vi "Write File Record.vi"(0 "MB session in":refnum<class "MB_Master.lvclass">, 1 "仪器版本":T1, 5 "File Number":u16, 7 "Record Number":u16, 9 "values":u16[](array[numeric]), 11 "error in (no error)":errorcluster) -> (4 "MB session out":refnum<class "MB_Master.lvclass">, 15 "error out":errorcluster)   [LabVIEW 2016, in "斯坦道总氮.lvlib"]
uses:
  <vilib>/Plasmionique/MB Master/MB_Master/MB_Master.lvclass
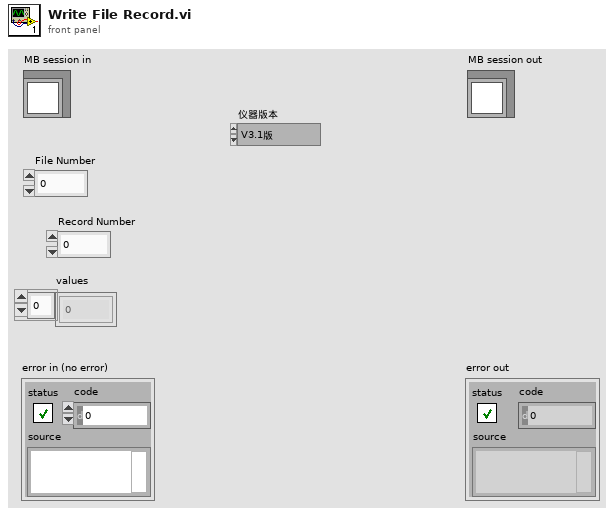
[diagram p1: front panel]
types:
  T1 = typedef "SingleStepTestV3.lvlib/SingleStepTestV3.lvclass/仪器版本.ctl" = enum16{"V3.1版", "V4版", "V3版", "V4.2版"}
  T2 = typedef "MB Master.lvlib/MB_PDU_Cluster.ctl" = cluster{"Function Code":u8, "Data":u8[], "RTU_DataBytes":i32}
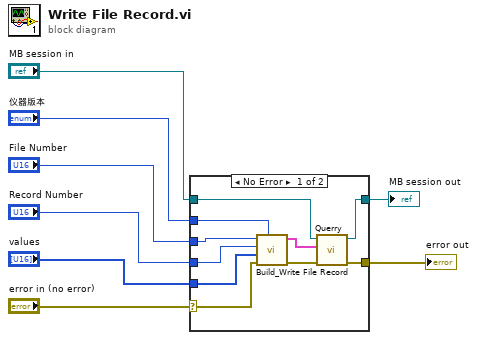
[diagram p0: block diagram]
diagram:
  n1 = case shown="No Error" "error in (no error)" {
    selector: "error in (no error)" -> [w13 w20]
    tunnel: [w17 w20] -> w7
    tunnel: [w18 w19] -> w5
    tunnel: "MB session in" -> [w16 w19]
    tunnel: "File Number" -> [w15 _]
    tunnel: "values" -> [w14 _]
    tunnel: "Record Number" -> [w10 _]
    tunnel: "仪器版本" -> [w9 _]
    frame No Error {
      n2 = call "Build_Write File Record.vi"("File Number"=w15, "Record Number"=w10, "values"=w14, "error in (no error)"=w13, "仪器版本"=w9) -> ("MB_PDU"=w12:T2, "error out"=w11:errorcluster)  [unwired: 4 in]
      n3 = call-dynamic "Querry.vi"("error in (no error)"=w11, "PDU_req"=w12, "MB_Master in"=w16) -> ("error out"=w17:errorcluster, "MB_Master out"=w18:refnum<class "MB_Master.lvclass">)  [unwired: 6 in, 1 out]
    }
    frame Error {
    }
  }
  "error out" <- w7
  "MB session out" <- w5
